vi "Enqueue Message (Single).vi"(6 "Priority Message? (F)":bool, 8 "error in (no error)":errorcluster, 9 "Message Data":variant, 10 "Message":string, 11 "Message Queue":refnum<queue>) -> (0 "error out":errorcluster, 3 "dup Message Queue":refnum<queue>)   [LabVIEW 2013, in "YKPZ400 Message Queue.lvlib"]
doc: "For a regular message, enqueue the message. For a priority message, enqueue it at the front of the queue."
uses:
  YKPZ400 Message Queue.lvlib
  Message Cluster.ctl
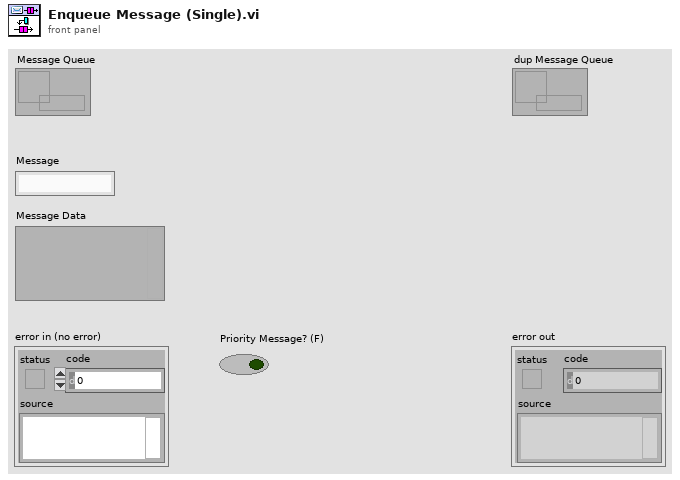
[diagram p1: front panel]
types:
  T1 = typedef "YKPZ400 Message Queue.lvlib/Message Cluster.ctl" = cluster{"Message":string, "Message Data":variant}
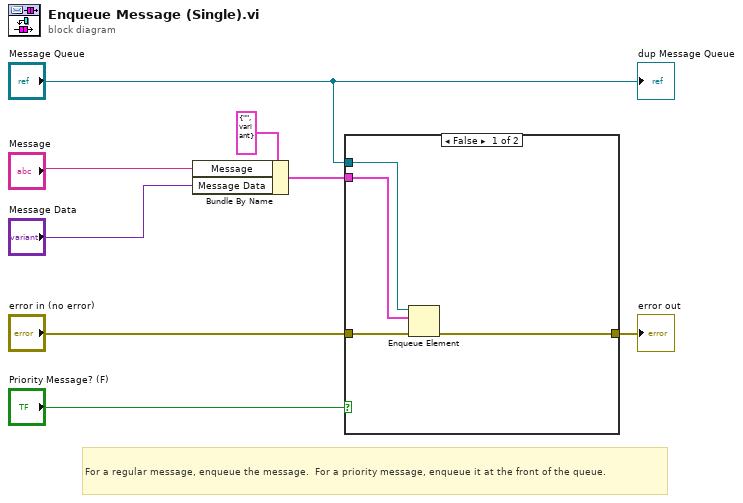
[diagram p0: block diagram]
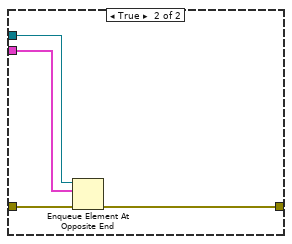
[diagram p2: hidden frame]
diagram:
  # "For a regular message, enqueue the message.  For a priority message, enqueue it at the front of the queue."
  n1 = Bundle By Name(cluster=T1 {"Message"="", "Message Data"=variant} ("Message Cluster"), "Message"="Message", "Message Data"="Message Data") -> (w1:T1)
  n2 = case shown="False" "Priority Message? (F)" {
    tunnel: "error in (no error)" -> [w12 w16]
    tunnel: [w11 w15] -> w3
    tunnel: "Message Queue" -> [w10 w14]
    tunnel: w1 -> [w9 w13]
    frame False {
      n3 = Enqueue Element(queue=w10, element=w9, error in (no error)=w12) -> (error out=w11:errorcluster)  [unwired: 1 in, 2 out]
    }
    frame True {
      n4 = Enqueue Element At Opposite End(queue=w14, element=w13, error in (no error)=w16) -> (error out=w15:errorcluster)  [unwired: 1 in, 2 out]
    }
  }
  "error out" <- w3
  "dup Message Queue" <- "Message Queue"
